vi "SP.vi"(6 "Valor":string, 8 "error in (no error)":errorcluster, 9 "Pin":u8, 10 "Puerto":u8, 11 "Serial Devices in":refnum<class "Serial Devices.lvclass">) -> (0 "error out":errorcluster, 3 "Serial Devices out":refnum<class "Serial Devices.lvclass">)   [LabVIEW 2019, in "Serial Devices.lvlib" / "Serial Devices.lvclass"]
uses:
  Serial Devices.lvclass
  C:/Program Files (x86)/National Instruments/LabVIEW 2019/vi.lib/ActorFramework/Actor/Actor.lvclass
  Serial Devices.lvclass/Serial Devices.ctl
  <vilib>/ActorFramework/Actor/Actor.lvclass/Actor.ctl
  <vilib>/ActorFramework/Message Enqueuer/Message Enqueuer.lvclass/Message Enqueuer.ctl
  NXP/NXP.lvclass
  TI/CYPRESS.lvclass
  SIMULATED/SIMULATED.lvclass
  <vilib>/ActorFramework/Message Enqueuer/Init from Existing Queue.vi
  <vilib>/ActorFramework/Message Enqueuer/Message Enqueuer.lvclass
  <vilib>/ActorFramework/Actor/Actor.lvclass
  Serial Devices.lvlib
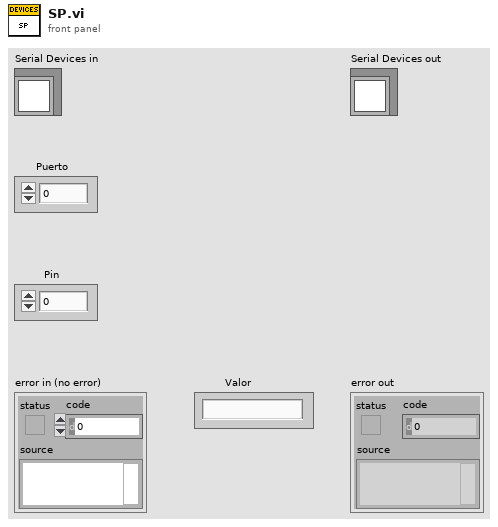
[diagram p1: front panel]
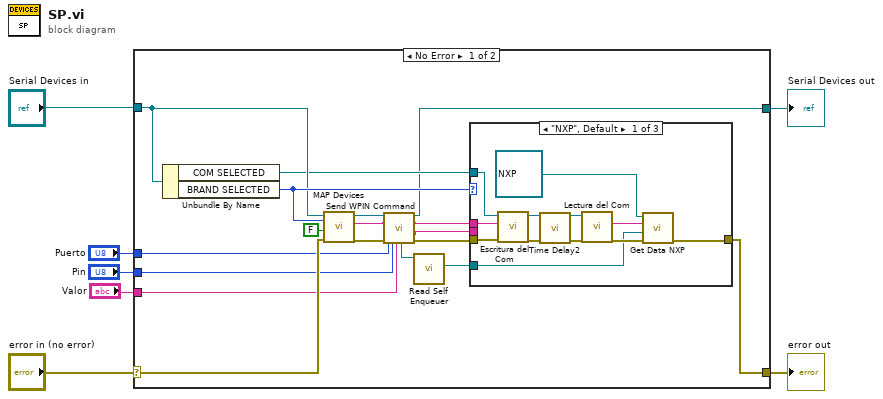
[diagram p0: block diagram]
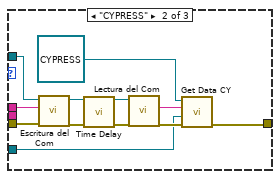
[diagram p2: hidden frame]
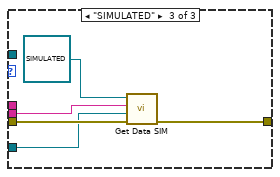
[diagram p3: hidden frame]
diagram:
  n1 = case shown="No Error" "error in (no error)" {
    selector: "error in (no error)" -> [w23 w53]
    tunnel: [w20 w53] -> w6
    tunnel: [w17 w52] -> w4
    tunnel: "Serial Devices in" -> [w19 w52]
    tunnel: "Puerto" -> [w9 _]
    tunnel: "Valor" -> [w10 _]
    tunnel: "Pin" -> [w8 _]
    frame No Error {
      n2 = Unbundle By Name(w19) -> ("COM SELECTED"=w18:refnum<visa-resource-name>, "BRAND SELECTED"=w22:enum16{"NXP", "CYPRESS", "SIMULATED"})
      n3 = call "MAP Devices.vi"("error in (no error)"=w23, "CREAR"=FALSE, "BRAND SELECTED"=w22, "Serial Devices in"=w19) -> ("error out"=w15:errorcluster, "VALOR"=w16:string, "Serial Devices out"=w11:refnum<class "Serial Devices.lvclass">)  [unwired: 5 in]
      n4 = call-dynamic "Send WPIN Command.vi"("Serial Devices in"=w11, "Device"=w16, "Puerto"=w9, "Pin"=w8, "error in"=w15, "Valor"=w10) -> ("Serial Devices out"=w17:refnum<class "Serial Devices.lvclass">, "Command"=w12:string, "Expected"=w13:string, "error out"=w14:errorcluster)  [unwired: 6 in]
      n5 = call <vilib>:"Read Self Enqueuer.vi"("Actor"=w11) -> ("Self Enqueuer"=w21:refnum<class "Message Enqueuer.lvclass">)  [unwired: 10 in]
      n6 = case shown="\"NXP\", Default" w22 {
        tunnel: w14 -> [w35 w46 w50]
        tunnel: w13 -> [_ _ w49]
        tunnel: w21 -> [w28 w39 w48]
        tunnel: [w27 w38 w47] -> w20
        tunnel: w18 -> [w33 w45 _]
        tunnel: w12 -> [w34 w44 _]
        frame "NXP", Default {
          n7 = call "Escritura del Com.vi"("error in (no error)"=w35, "write buffer"=w34, "VISA Refnum in"=w33) -> ("error out"=w26:errorcluster, "VISA resource name out"=w32:refnum<visa-resource-name>)  [unwired: 7 in]
          n8 = call "Time Delay2"("error in (no error)"=w26) -> ("error out"=w25:errorcluster)  [unwired: 10 in]
          n9 = call "Lectura del Com.vi"("error in (no error)"=w25, "VISA Refnum in"=w32) -> ("error out"=w29:errorcluster, "Serial Response"=w30:string)  [unwired: 7 in, 1 out]
          n10 = call "Get Data NXP.vi"("error in"=w29, "Data Enqueuer"=w28, "Data"=w30, "NXP in"=refnum<class "NXP.lvclass"> refnum ("NXP.lvclass")) -> ("error out"=w27:errorcluster)  [unwired: 6 in, 1 out]
        }
        frame "CYPRESS" {
          n11 = call "Escritura del Com.vi"("error in (no error)"=w46, "write buffer"=w44, "VISA Refnum in"=w45) -> ("error out"=w37:errorcluster, "VISA resource name out"=w43:refnum<visa-resource-name>)  [unwired: 7 in]
          n12 = call "Time Delay"("error in (no error)"=w37) -> ("error out"=w36:errorcluster)  [unwired: 10 in]
          n13 = call "Lectura del Com.vi"("error in (no error)"=w36, "VISA Refnum in"=w43) -> ("error out"=w40:errorcluster, "Serial Response"=w41:string)  [unwired: 7 in, 1 out]
          n14 = call "Get Data CY.vi"("error in"=w40, "Data Enqueuer"=w39, "Data"=w41, "CYPRESS in"=refnum<class "CYPRESS.lvclass"> refnum ("CYPRESS.lvclass")) -> ("error out"=w38:errorcluster)  [unwired: 6 in, 1 out]
        }
        frame "SIMULATED" {
          n15 = call "Get Data SIM.vi"("error in"=w50, "Data Enqueuer"=w48, "Data"=w49, "SIMULATED in"=refnum<class "SIMULATED.lvclass"> refnum ("SIMULATED.lvclass")) -> ("error out"=w47:errorcluster)  [unwired: 6 in, 1 out]
        }
      }
    }
    frame Error {
    }
  }
  "error out" <- w6
  "Serial Devices out" <- w4
